vi "Update Acquisition Settings Msg.vi"(8 "error in (no error)":errorcluster, 10 "Config":T4={"Hardware Configuration"={"COM Port"="", "Reference Distance"=0.0, "Sensor SN"=""}, "Logging Configuration"={"Log File Base Path"=path "", "Datafile Ref"=refnum, "Database Ref"=refnum}, "UI Refs"={"Start Ref"=refnum, "Settings Ref"=refnum, "Stop Ref"=refnum, "Exit Ref"=refnum, "Status Ref"=refnum, "Data Ref"=refnum, "StatusBox Ref"=refnum, "Location Ref"=refnum, "Operator Ref"=refnum, "Time Ref"=refnum, "Test in Progess Ref"=refnum}, "Calibration Data"={"calibrationID"=0, "operatorID"=0, "sensorID"=0, "start_time"="", "end_time"="", "offset"=0.0, "offset_units"="", "ring_time"=0.0, "error"=0.0, "Passed"=0, "data_storage_location"="", "comments"=""}, "Time Elapsed"=0, "Samples Required"=480} {"Hardware Configuration"."Reference Distance" format="%.3g"}, 11 "Message Queues in":T1) -> (0 "error out":errorcluster, 3 "Message Queues out":T1)   [LabVIEW 2018, in "Acquisition.lvlib"]
uses:
  Acquisition.lvlib
  Settings/Settings.ctl
  Hardware Configuration.ctl
  Logging/Logging Configuration.ctl
  <vilib>/addons/database/Connection.llb/Conn ObjectReference.ctl
  Controls/Location Ring.ctl
  Controls/Time Remaining.ctl
  Support/Message Queue/All Message Queues.ctl
  Support/Message Queue/Message Cluster.ctl
  Controls/Data Queue.ctl
  Controls/Acquired Data.ctl
  Controls/Data Notifier.ctl
  Support/Message Queue/Enqueue Message (Single).vi
  support/Message Queue/Message Queue.lvlib
  <vilib>/addons/database/NI_Database_API.lvlib
  Logging/Logging.lvlib
  Settings/Settings.lvlib
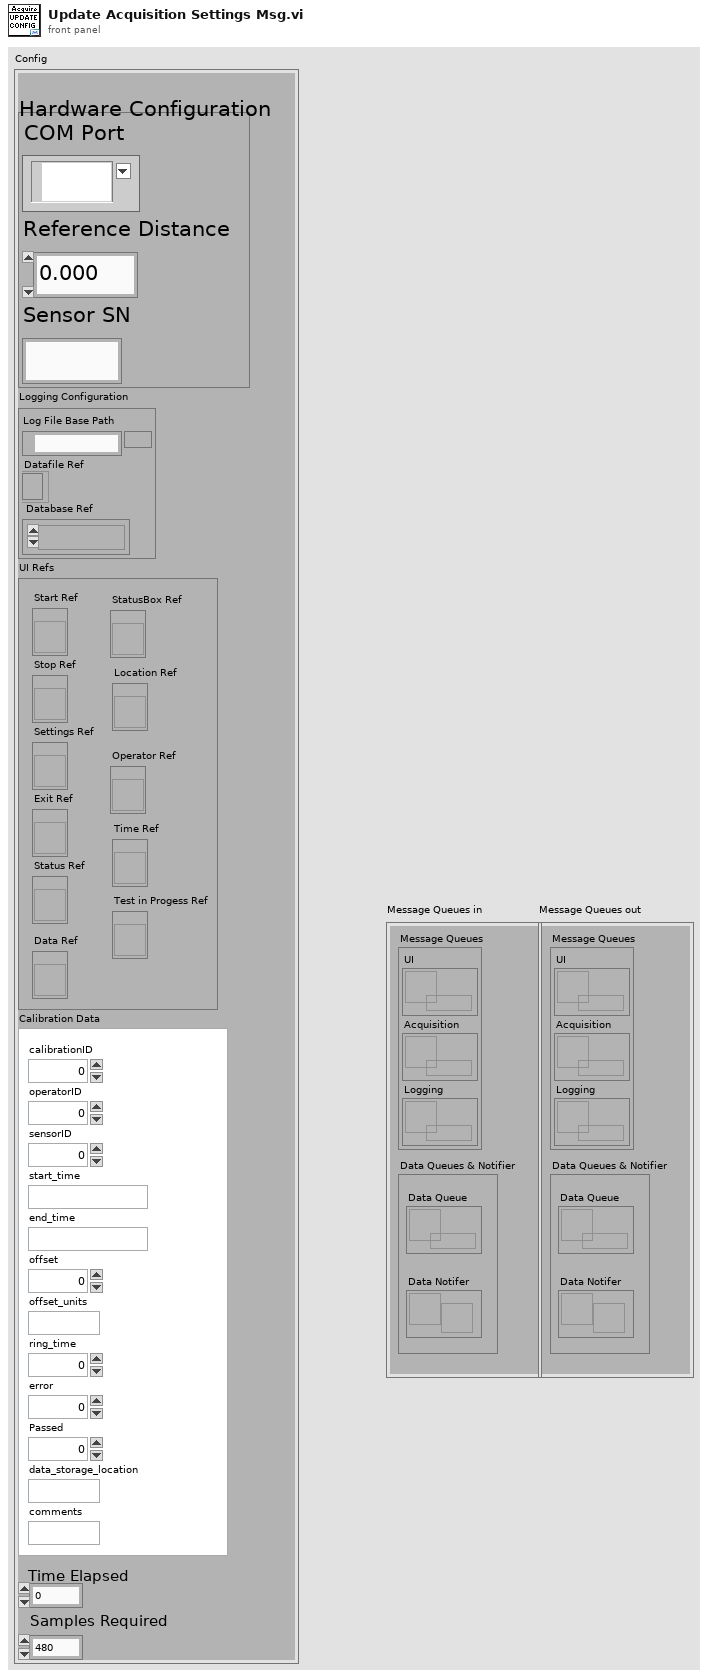
[diagram p1: front panel]
types:
  T1 = typedef "Message Queue.lvlib/All Message Queues.ctl" = cluster{"Message Queues":cluster{"UI":refnum<queue>, "Acquisition":refnum<queue>, "Logging":refnum<queue>}, "Data Queues & Notifier":cluster{"Data Queue":T2, "Data Notifer":T3}}
  T2 = typedef "Data Queue.ctl" = refnum<queue>
  T3 = typedef "Data Notifier.ctl" = refnum<notifier>
  T4 = typedef "Settings.lvlib/Settings.ctl" = cluster{"Hardware Configuration":T5, "Logging Configuration":T6, "UI Refs":cluster{"Start Ref":refnum<vi>, "Settings Ref":refnum<vi>, "Stop Ref":refnum<vi>, "Exit Ref":refnum<vi>, "Status Ref":refnum<vi>, "Data Ref":refnum<vi>, "StatusBox Ref":refnum<vi>, "Location Ref":refnum<vi>, "Operator Ref":refnum<vi>, "Time Ref":refnum<vi>, "Test in Progess Ref":refnum<vi>}, "Calibration Data":cluster{"calibrationID":u16, "operatorID":u16, "sensorID":u16, "start_time":string, "end_time":string, "offset":dbl, "offset_units":string, "ring_time":dbl, "error":dbl, "Passed":u8, "data_storage_location":string, "comments":string}, "Time Elapsed":u16, "Samples Required":u16}
  T5 = typedef "Acquisition.lvlib/Hardware Configuration.ctl" = cluster{"COM Port":refnum<visa-resource-name>, "Reference Distance":dbl, "Sensor SN":string}
  T6 = typedef "Logging.lvlib/Logging Configuration.ctl" = cluster{"Log File Base Path":path, "Datafile Ref":refnum<file>, "Database Ref":T7}
  T7 = typedef "NI_Database_API.lvlib/Conn ObjectReference.ctl" = refnum<k1>
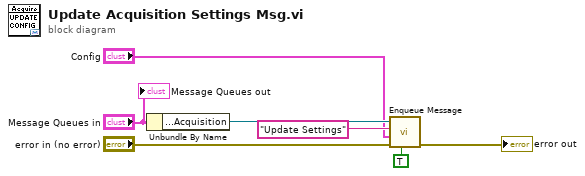
[diagram p0: block diagram]
diagram:
  n1 = Unbundle By Name("Message Queues in") -> ("Message Queues.Acquisition"=w2:refnum<queue>)
  n2 = call-poly "Enqueue Message.vi"("Priority Message? (F)"=TRUE, "error in (no error)"="error in (no error)", "Message Data"="Config", "Message"="Update Settings", "Message Queue"=w2) -> ("error out"=→"error out":errorcluster)  [unwired: 5 in, 1 out]
  "Message Queues out" <- "Message Queues in"
